vi "EXAMPLE - ConfigSampleRate.vi"(8 "Fehler (Eingang, kein Fehler)":errorcluster, 11 "IP":string) -> (0 "error out":errorcluster)   [LabVIEW 2016]
uses:
  <vilib>/Utility/config.llb/Write Key (String).vi
  <vilib>/Utility/config.llb/Read Key (Double).vi
  <vilib>/Utility/config.llb/NI_LVConfig.lvlib
panel:
  in  "OK-Schaltfläche":bool
  in  "New Frequency":string
  in  "EXIT":bool
  out "Sample frequency":dbl caption="Actual Frequency" format="%.2f"
  # "Configure sample rate"
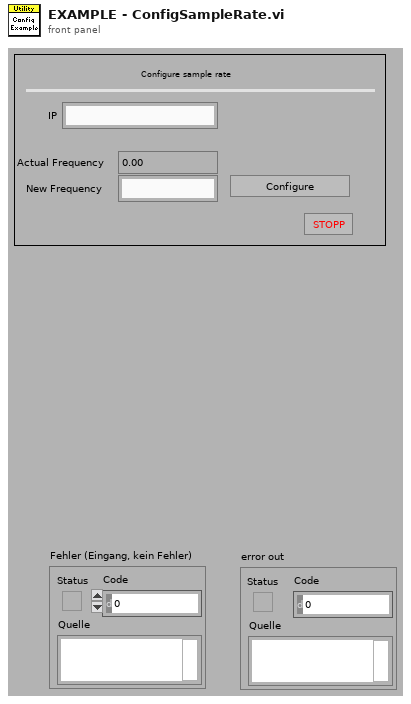
[diagram p1: front panel]
types:
  T1 = enum16{"Supervisor", "Configuration", "Datatransfer"}
  T2 = typedef "NI_LVConfig.lvlib/Config Data RefNum.ctl" = refnum<k1>
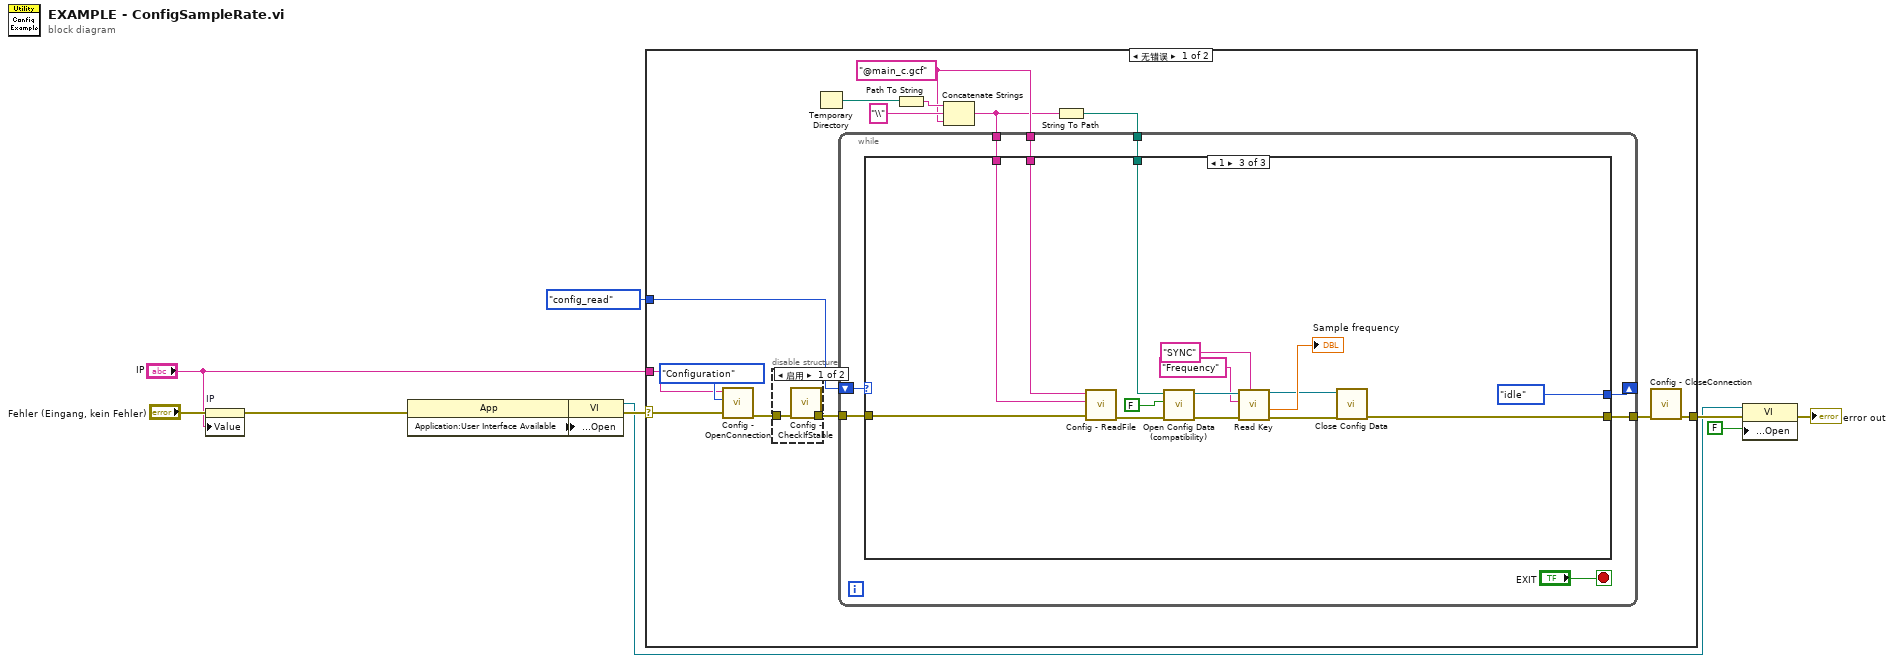
[diagram p0: block diagram]
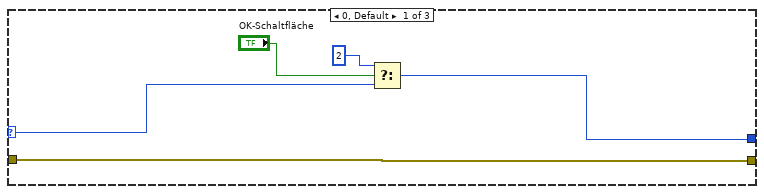
[diagram p3: hidden frame]
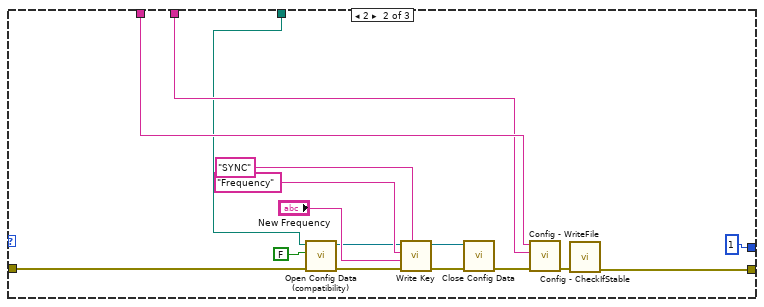
[diagram p4: hidden frame]
diagram:
  n1 = property on="IP" class="Str"(error in="Fehler (Eingang, kein Fehler)", "Value"="IP") -> (error out=w3:errorcluster)  [unwired: 1 in, 1 out]
  n2 = property class="App"(error in=w3) -> (error out=w9:errorcluster, "Application:User Interface Available"=w10:bool)  [unwired: 1 in, 1 out]
  n3 = property class="VI"(error in=w9, "Front Panel.Open"=w10) -> (reference out=w4:refnum<vi>, error out=w5:errorcluster)  [unwired: 1 in]
  n4 = case shown="无错误" w5 {
    selector: w5 -> [w15 w73]
    tunnel: "IP" -> [w12 _]
    tunnel: enum16{"idle", "config_read", "config_write"}."config_read" ("State") -> [w13 _]
    tunnel: [w18 w73] -> w7
    frame No Error {
      w21 = "@main_c.gcf" ("SourceFileName")
      n5 = call "Config - OpenConnection.vi"("Fehler (Eingang, kein Fehler)"=w15, "Mode"=T1."Configuration", "IP/DNS"=w12) -> ("Fehler (Ausgang)"=w16:errorcluster)  [unwired: 8 out]
      n6 = disable-structure shown="启用" {
        disable-tunnel: w16 -> [w27 w28]
        disable-tunnel: [w26 w28] -> w14
        frame Enabled {
          n7 = call "Config - CheckIfStable.vi"("Fehler (Eingang, kein Fehler)"=w27) -> ("Fehler (Ausgang)"=w26:errorcluster)  [unwired: 10 out]
        }
        frame Disabled {
        }
      }
      n8 = Temporary Directory() -> (w24:path)
      n9 = Path To String(path=w24) -> (string=w25:string)
      n10 = Concatenate Strings(w25, "\\" ("DestinationFullFileName"), w21) -> (w20:string)
      n11 = String To Path(string=w20) -> (path=w22:path)
      n12 = while {
        tunnel: w14 -> [w36]
        shift-right: [w33] -> _
        shift-left: w13 -> [w34]
        tunnel: w21 -> [w32]
        tunnel: w20 -> [w31]
        tunnel: w22 -> [w30]
        tunnel: [w29] -> w19
        stop <- "EXIT" stop-if-true
        n13 = case shown="1" w34 {
          selector: w34 -> [w41 _ _]
          tunnel: w36 -> [w37 w42 w58]
          tunnel: [w38 u16 1 ("t") enum16{"idle", "config"}."idle" ("State")] -> w33
          tunnel: w32 -> [_ w54 w63]
          tunnel: w31 -> [_ w55 w64]
          tunnel: w30 -> [_ w43 w62]
          tunnel: [w37 w53 w59] -> w29
          frame 0, Default {
            n14 = Select(t=u16 2, s="OK-Schaltfläche", f=w41) -> (s? t:f=w38:u16)
          }
          frame 2 {
            n15 = call <vilib>:"Open Config Data (compatibility).vi"("error in (no error)"=w42, "create file if necessary (T)"=FALSE ("create file if necessary? (T)"), "configuration file path"=w43) -> ("error out"=w48:errorcluster, "refnum"=w44:T2)  [unwired: 6 in, 1 out]
            n16 = call-poly <vilib>:"Write Key.vi"("section"="SYNC", "error in (no error)"=w48, "value"="New Frequency", "key"="Frequency", "refnum"=w44) -> ("error out"=w50:errorcluster, "refnum out"=w49:T2)  [unwired: 1 in, 4 out]
            n17 = call <vilib>:"Close Config Data.vi"("error in (no error)"=w50, "refnum"=w49) -> ("error out"=w51:errorcluster)  [unwired: 1 in, 8 out]
            n18 = call "Config - WriteFile.vi"("Fehler (Eingang, kein Fehler)"=w51, "DestinationFileName"=w54, "SourceFullFileName"=w55) -> ("Fehler (Ausgang)"=w56:errorcluster)  [unwired: 8 out]
            n19 = call "Config - CheckIfStable.vi"("Fehler (Eingang, kein Fehler)"=w56) -> ("Fehler (Ausgang)"=w53:errorcluster)  [unwired: 10 out]
          }
          frame 1 {
            n20 = call "Config - ReadFile.vi"("Fehler (Eingang, kein Fehler)"=w58, "DestinationFullFileName"=w64, "SourceFileName"=w63) -> ("Fehler (Ausgang)"=w72:errorcluster)  [unwired: 8 out]
            n21 = call <vilib>:"Open Config Data (compatibility).vi"("error in (no error)"=w72, "create file if necessary (T)"=FALSE ("create file if necessary? (T)"), "configuration file path"=w62) -> ("error out"=w70:errorcluster, "refnum"=w68:T2)  [unwired: 6 in, 1 out]
            n22 = call-poly <vilib>:"Read Key.vi"("section"="SYNC", "error in (no error)"=w70, "key"="Frequency", "refnum"=w68) -> ("error out"=w60:errorcluster, "value"=→"Sample frequency":dbl, "refnum out"=w61:T2)  [unwired: 1 in, 4 out]
            n23 = call <vilib>:"Close Config Data.vi"("error in (no error)"=w60, "refnum"=w61) -> ("error out"=w59:errorcluster)  [unwired: 1 in, 8 out]
          }
        }
      }
      n24 = call "Config - CloseConnection.vi"("Fehler (Eingang, kein Fehler)"=w19) -> ("Fehler (Ausgang)"=w18:errorcluster)  [unwired: 10 out]
    }
    frame Error {
    }
  }
  n25 = property class="VI"(reference=w4, error in=w7, "Front Panel.Open"=FALSE ("Frontpanel-Fenster:Öffnen")) -> (error out=→"error out":errorcluster)  [unwired: 1 out]
